vi "Start livestream video from CamServer (TCP CLIENT).vi"(4 "Quality":i32=750 min=0 max=1000, 6 "Resolution":T1 items=["Low", "Med.", "High", "Max."], 7 "Camera":T3="Travcam", 8 "Video name":string, 9 "Video directory path":path, 10 "Write video":bool, 11 "TCP/IP port":u16=80) -> (0 "Error out":errorcluster)   [LabVIEW 2016]
doc: "Starts a video livestream from the camera server. The stream can also be saved to a local directory."
uses:
  Camera enum/Camera enum.ctl
  Camera enum/Camera resolution.ctl
  Anemometry/Anemometry Sub Vis/File/Setup_Filetype.ctl
  <vilib>/vision/Avi.llb/IMAQ AVI2 Refnum.ctl
  Globals/CamServer global.vi
panel:
  in  "Crosshair color":u32(colorbox)=16711935
  in  "Show crosshair":bool=TRUE
  in  "Stop":bool
  out "Video":T2(plugin-control)
  # "PN 25/08/15"
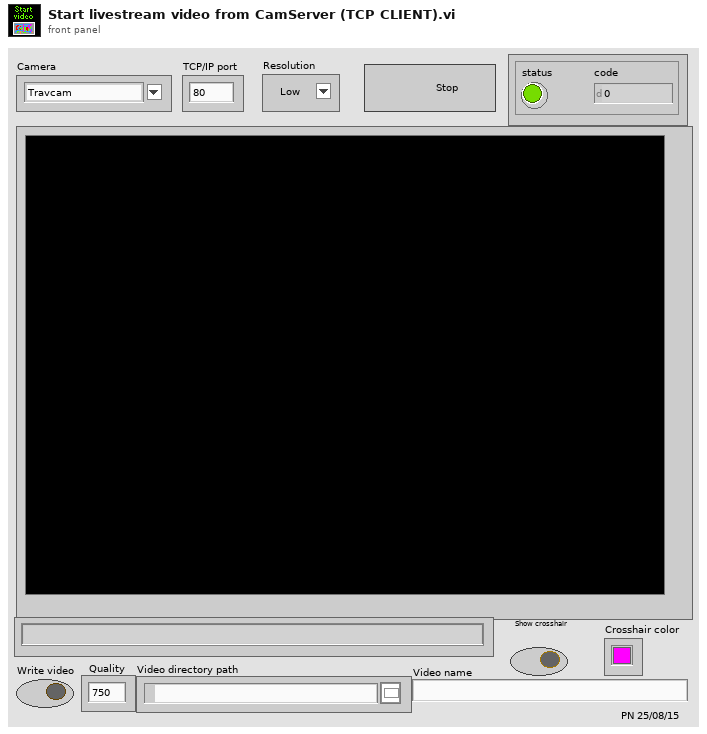
[diagram p1: front panel]
types:
  T1 = typedef "Camera resolution.ctl" = u8
  T2 = typedef "IMAQ Image.ctl" = refnum<image>
  T3 = typedef "Camera enum.ctl" = string
  T4 = typedef "Setup_Filetype.ctl" = enum16{"Measurement Setups", "Calibration Setups", "General", "Results File Plotter Setups", "Speed Calib Tweaks"}
  T5 = typedef "IMAQ AVI2 Refnum.ctl" = refnum<k20>
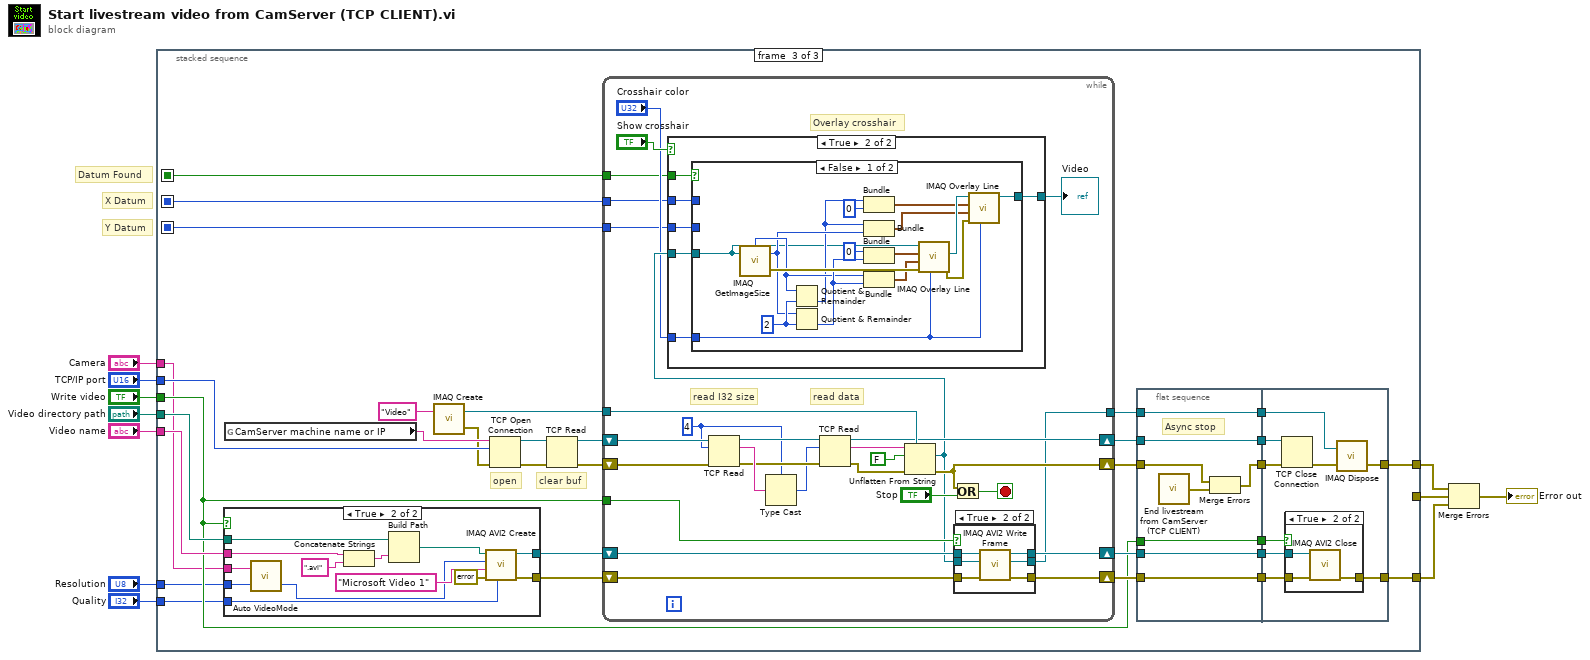
[diagram p0: block diagram]
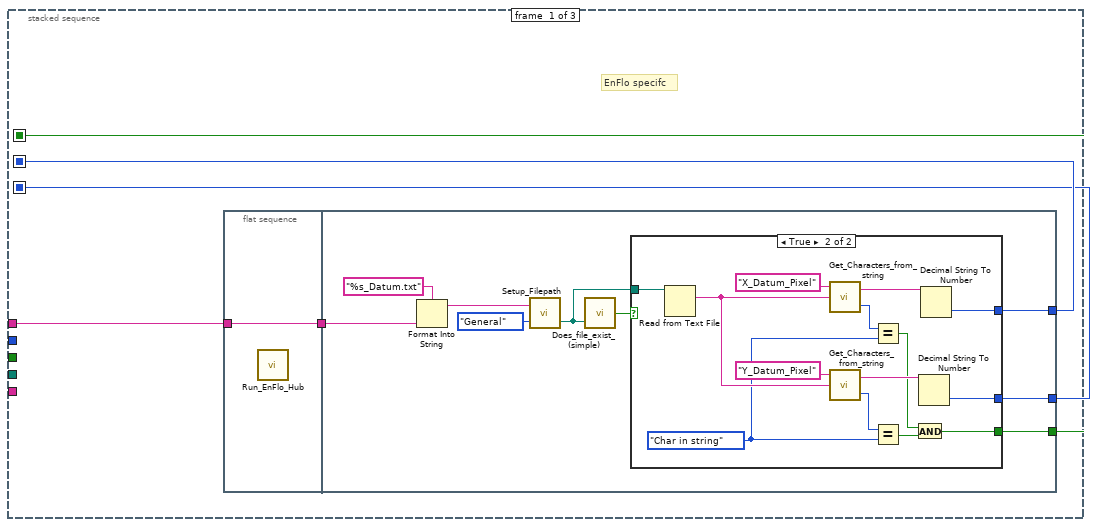
[diagram p2: hidden frame]
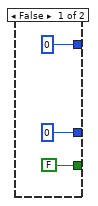
[diagram p3: hidden frame]
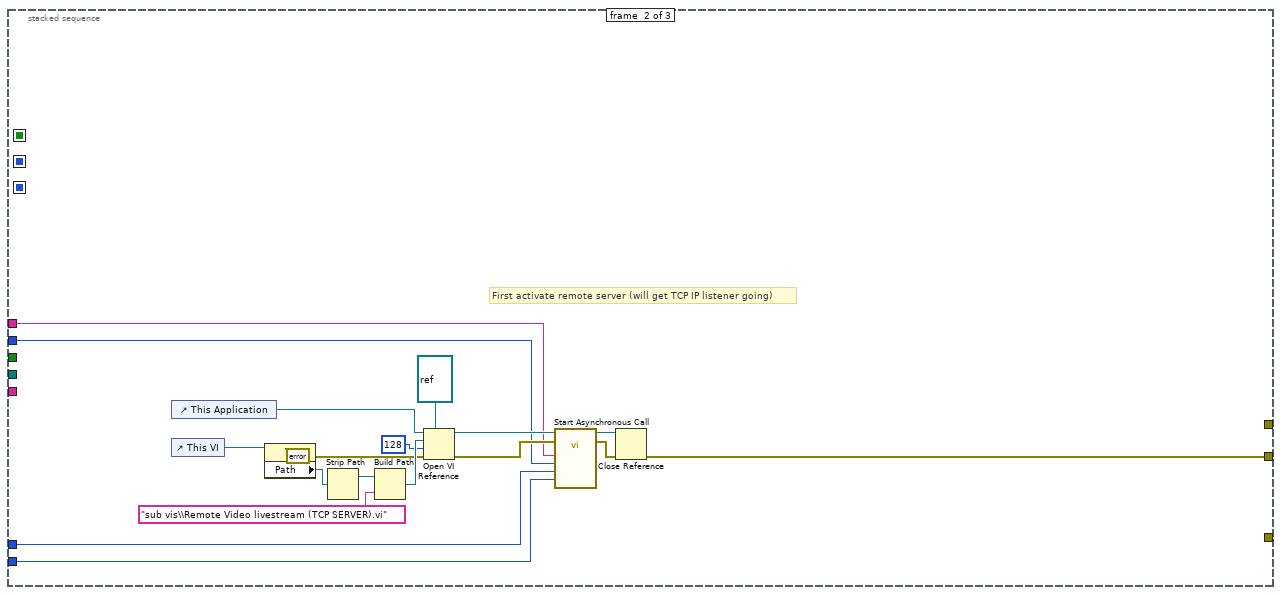
[diagram p4: hidden frame]
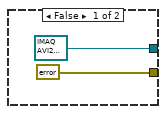
[diagram p5: hidden frame]
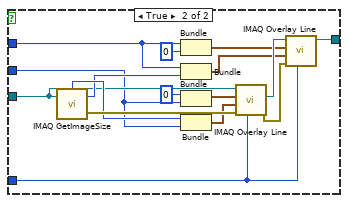
[diagram p8: hidden frame]
diagram:
  # "Datum Found"
  # "Y Datum"
  # "X Datum"
  n1 = stacked-sequence {
    seq-local: [w15 _ _] -> [_ _ w66]
    seq-local: [w14 _ _] -> [_ _ w65]
    seq-local: [w13 _ _] -> [_ _ w67]
    tunnel: "Camera" -> [w16 w48 w64]
    tunnel: "TCP/IP port" -> [_ w47 w95]
    tunnel: "Write video" -> [_ _ w70]
    tunnel: [_ w46 _] -> w8
    tunnel: [_ _ w80] -> w7
    tunnel: [_ _ w73] -> w5
    tunnel: "Video name" -> [_ _ w72]
    tunnel: "Video directory path" -> [_ _ w71]
    tunnel: "Quality" -> [_ w45 w68]
    tunnel: "Resolution" -> [_ w44 w63]
    frame #0 {
      # "EnFlo specifc"
      n2 = flat-sequence {
        tunnel: w16 -> [w17]
        tunnel: [w17] -> w12
        tunnel: [w20] -> w15
        tunnel: [w19] -> w14
        tunnel: [w18] -> w13
        tunnel: w12 -> [w25]
        frame #0 {
          n3 = call "Run_EnFlo_Hub.vi"() -> ()  [unwired: 7 in, 1 out]
        }
        frame #1 {
          n4 = Format Into String(format string="%s_Datum.txt", w25) -> (resulting string=w23:string)  [unwired: 2 in, 1 out]
          n5 = call "Setup_Filepath.vi"("Setup File Type"=Setup_Filetype."General", "Filename in"=w23) -> ("Filename Out"=w21:path)  [unwired: 1 out]
          n6 = call "Does_file_exist_(simple).vi"("Pathname"=w21) -> ("exists?"=w22:bool)
          n7 = case shown="True" w22 {
            tunnel: w21 -> [_ w43]
            tunnel: [0 w40] -> w20
            tunnel: [0 w36] -> w19
            tunnel: [FALSE w30] -> w18
            frame False {
            }
            frame True {
              w35 = enum16{"Char in string", "Char not in string"}."Char in string" ("Status")
              n8 = Read from Text File(file (use dialog)=w43) -> (text=w37:string)  [unwired: 3 in, 3 out]
              n9 = call "Get_Characters_from_string.vi"("Input string"=w37, "Variable name"="X_Datum_Pixel") -> ("Status"=w34:enum16{"Char in string", "Char not in string"}, "Value"=w41:string)  [unwired: 1 in]
              n10 = call "Get_Characters_from_string.vi"("Input string"=w37, "Variable name"="Y_Datum_Pixel") -> ("Status"=w33:enum16{"Char in string", "Char not in string"}, "Value"=w39:string)  [unwired: 1 in]
              n11 = Equal?(x=w34, y=w35) -> (x = y?=w31:bool)
              n12 = Equal?(x=w33, y=w35) -> (x = y?=w32:bool)
              n13 = And(x=w31, y=w32) -> (x .and. y?=w30:bool)
              n14 = Decimal String To Number(string=w39) -> (number=w36:i32)  [unwired: 2 in, 1 out]
              n15 = Decimal String To Number(string=w41) -> (number=w40:i32)  [unwired: 2 in, 1 out]
            }
          }
        }
      }
    }
    frame #1 {
      # "First activate remote server (will get TCP IP listener going)"
      n16 = control-ref of="This Application"() -> (w57:refnum<vi>)
      n17 = control-ref of="This VI"() -> (w62:refnum<vi>)
      n18 = property class="VI"(reference=w62, error in=errorcluster {"status"=FALSE, "code"=0, "source"=""} ("error in (no error)")) -> (error out=w59:errorcluster, "Path"=w55:path)  [unwired: 1 out]
      n19 = Strip Path(path=w55) -> (stripped path=w54:path)  [unwired: 1 out]
      n20 = Build Path(base path=w54, name or relative path="sub vis\\Remote Video livestream (TCP SERVER).vi") -> (appended path=w60:path)
      n21 = Open VI Reference(type specifier VI Refnum (for type only)=refnum<vi> refnum, application reference (local)=w57, vi path=w60, options=128, error in (no error)=w59) -> (vi reference=w53:refnum<vi>, error out=w52:errorcluster)  [unwired: 1 in]
      n22 = call-by-ref "Start Asynchronous Call"(reference=w53, error in=w52, "Quality"=w45, "Resolution"=w44, "TCP/IP port"=w47, "Camera"=w48) -> (reference out=w50:refnum<vi>, error out=w49:errorcluster)  [unwired: 1 out]
      n23 = Close Reference(reference=w50, error in (no error)=w49) -> (error out=w46:errorcluster)
    }
    frame #2 {
      # "open"
      # "clear buf"
      n24 = case shown="True" w70 {
        tunnel: [T5 refnum ("AVI Refnum") w110] -> w79
        tunnel: [errorcluster {"status"=FALSE, "code"=0, "source"=""} ("error out") w109] -> w78
        tunnel: w72 -> [_ w103]
        tunnel: w71 -> [_ w102]
        tunnel: w68 -> [_ w101]
        tunnel: w64 -> [_ w100]
        tunnel: w63 -> [_ w99]
        frame False {
        }
        frame True {
          n25 = call "Auto VideoMode.vi"("Resolution"=w99, "Camera"=w100) -> ("FPS"=w98:u32)  [unwired: 1 out]
          n26 = Concatenate Strings(w103, ".avi" ("name or relative path")) -> (w105:string)
          n27 = Build Path(base path=w102, name or relative path=w105) -> (appended path=w104:path)
          n28 = call "IMAQ AVI2 Create"("Quality"=w101, "error in (no error)"=errorcluster {"status"=FALSE, "code"=0, "source"=""} ("error in"), "Codec"="Microsoft Video 1", "Frames Per Second"=w98, "AVI Path"=w104) -> ("error out"=w109:errorcluster, "AVI Refnum"=w110:T5)  [unwired: 5 in]
        }
      }
      n29 = global read "CamServer global.vi" "CamServer machine name or IP"() -> (w94:string)
      n30 = call "IMAQ Create"("Image Name"="Video") -> ("New Image"=w88:T2, "error out"=w87:errorcluster)  [unwired: 4 in]
      n31 = TCP Open Connection(address=w94, remote port or service name=w95, error in (no error)=w87) -> (connection ID=w92:refnum<k5>, error out=w93:errorcluster)  [unwired: 2 in]
      n32 = TCP Read(connection ID=w92, error in (no error)=w93) -> (connection ID out=w90:refnum<k5>, error out=w91:errorcluster)  [unwired: 3 in, 1 out]
      n33 = while {
        shift-right: [w148] -> w86
        shift-left: w90 -> [w159]
        shift-right: [w147] -> w85
        shift-left: w91 -> [w157]
        tunnel: w88 -> [w150]
        tunnel: [w139] -> w84
        shift-right: [w142] -> w74
        shift-left: w78 -> [w141]
        shift-right: [w143] -> w77
        shift-left: w79 -> [w144]
        tunnel: w70 -> [w140]
        tunnel: w67 -> [w134]
        tunnel: w66 -> [w133]
        tunnel: w65 -> [w132]
        stop <- w145 stop-if-true
        w149 = 4
        # "Overlay crosshair"
        # "read data"
        # "read I32 size"
        n34 = TCP Read(connection ID=w159, bytes to read=w149, error in (no error)=w157) -> (connection ID out=w156:refnum<k5>, data out=w158:string, error out=w155:errorcluster)  [unwired: 2 in]
        n35 = Type Cast(type=w149, x=w158) -> (*(type *) &x=w154:i32)
        n36 = TCP Read(connection ID=w156, bytes to read=w154, error in (no error)=w155) -> (connection ID out=w148:refnum<k5>, data out=w153:string, error out=w151:errorcluster)  [unwired: 2 in]
        n37 = Unflatten From String(type=w150, binary string=w153, data includes array or string size? (T)=FALSE, error in (no error)=w151) -> (value=w137:T2, error out=w147:errorcluster)  [unwired: 1 in, 1 out]
        n38 = case shown="True" "Show crosshair" {
          tunnel: [w160 w166] -> w138
          tunnel: w137 -> [w160 w165]
          tunnel: "Crosshair color" -> [_ w164]
          tunnel: w134 -> [_ w163]
          tunnel: w133 -> [_ w162]
          tunnel: w132 -> [_ w161]
          frame False {
          }
          frame True {
            n39 = case shown="False" w163 {
              tunnel: [w175 w193] -> w166
              tunnel: w165 -> [w168 w187]
              tunnel: w164 -> [w167 w186]
              tunnel: w162 -> [_ w185]
              tunnel: w161 -> [_ w184]
              frame False {
                w182 = 2 ("y")
                n40 = call "IMAQ GetImageSize"("Image"=w168) -> ("Y Resolution"=w170:i32, "X Resolution"=w177:i32, "error out"=w183:errorcluster)  [unwired: 3 in]
                n41 = Quotient & Remainder(x=w177, y=w182) -> (floor(x/y)=w169:i32)  [unwired: 1 out]
                n42 = Quotient & Remainder(x=w170, y=w182) -> (floor(x/y)=w179:i32)  [unwired: 1 out]
                n43 = Bundle(w169, "y"=0) -> (w173:cluster{i32, "y":i32})  [unwired: 1 in]
                n44 = Bundle(w169, "Y Resolution"=w170) -> (w172:cluster{i32, "Y Resolution":i32})  [unwired: 1 in]
                n45 = Bundle("y"=0, w179) -> (w181:cluster{"y":i32, i32})  [unwired: 1 in]
                n46 = Bundle("X Resolution"=w177, w179) -> (w180:cluster{"X Resolution":i32, i32})  [unwired: 1 in]
                n47 = call "IMAQ Overlay Line"("Color"=w167, "error in (no error)"=w183, "End Point"=w180, "Start Point"=w181, "Image"=w168) -> ("error out"=w174:errorcluster, "Image Out"=w176:T2)  [unwired: 5 in]
                n48 = call "IMAQ Overlay Line"("Color"=w167, "error in (no error)"=w174, "End Point"=w172, "Start Point"=w173, "Image"=w176) -> ("Image Out"=w175:T2)  [unwired: 5 in, 1 out]
              }
              frame True {
                n49 = call "IMAQ GetImageSize"("Image"=w187) -> ("Y Resolution"=w188:i32, "X Resolution"=w195:i32, "error out"=w199:errorcluster)  [unwired: 3 in]
                n50 = Bundle(w185, "y"=0) -> (w191:cluster{i32, "y":i32})  [unwired: 1 in]
                n51 = Bundle(w185, "Y Resolution"=w188) -> (w190:cluster{i32, "Y Resolution":i32})  [unwired: 1 in]
                n52 = Bundle("y"=0, w184) -> (w198:cluster{"y":i32, i32})  [unwired: 1 in]
                n53 = Bundle("X Resolution"=w195, w184) -> (w197:cluster{"X Resolution":i32, i32})  [unwired: 1 in]
                n54 = call "IMAQ Overlay Line"("Color"=w186, "error in (no error)"=w199, "End Point"=w197, "Start Point"=w198, "Image"=w187) -> ("error out"=w192:errorcluster, "Image Out"=w194:T2)  [unwired: 5 in]
                n55 = call "IMAQ Overlay Line"("Color"=w186, "error in (no error)"=w192, "End Point"=w190, "Start Point"=w191, "Image"=w194) -> ("Image Out"=w193:T2)  [unwired: 5 in, 1 out]
              }
            }
          }
        }
        "Video" <- w138
        n56 = Or(x=w147, y="Stop") -> (x .or. y?=w145:bool)
        n57 = case shown="True" w140 {
          tunnel: w144 -> [w202 w208]
          tunnel: w137 -> [w200 w207]
          tunnel: [w202 w206] -> w143
          tunnel: [w201 w205] -> w142
          tunnel: w141 -> [w201 w204]
          tunnel: [w200 w203] -> w139
          frame False {
          }
          frame True {
            n58 = call "IMAQ AVI2 Write Frame"("error in (no error)"=w204, "Image"=w207, "AVI Refnum"=w208) -> ("error out"=w205:errorcluster, "Image Out (duplicate)"=w203:T2, "AVI Refnum (duplicate)"=w206:T5)  [unwired: 6 in]
          }
        }
      }
      n59 = flat-sequence {
        tunnel: w84 -> [w117]
        tunnel: w85 -> [w115]
        tunnel: w86 -> [w118]
        tunnel: [w118] -> w83
        tunnel: [w114] -> w82
        tunnel: [w117] -> w81
        tunnel: w77 -> [w113]
        tunnel: [w113] -> w76
        tunnel: w74 -> [w112]
        tunnel: [w112] -> w75
        tunnel: w70 -> [w111]
        tunnel: [w111] -> w69
        tunnel: w83 -> [w127]
        tunnel: w82 -> [w126]
        tunnel: w81 -> [w124]
        tunnel: [w123] -> w80
        tunnel: w76 -> [w122]
        tunnel: w75 -> [w121]
        tunnel: [w120] -> w73
        tunnel: w69 -> [w119]
        frame #0 {
          # "Async stop"
          n60 = call "End livestream from CamServer (TCP CLIENT).vi"() -> ("Error out"=w116:errorcluster)  [unwired: 1 in]
          n61 = Merge Errors(w115, w116) -> (w114:errorcluster)
        }
        frame #1 {
          n62 = TCP Close Connection(connection ID=w127, error in (no error)=w126) -> (error out=w125:errorcluster)  [unwired: 1 in, 1 out]
          n63 = case shown="True" w119 {
            tunnel: w121 -> [w128 w131]
            tunnel: [w128 w130] -> w120
            tunnel: w122 -> [_ w129]
            frame False {
            }
            frame True {
              n64 = call "IMAQ AVI2 Close"("error in (no error)"=w131, "AVI Refnum"=w129) -> ("error out"=w130:errorcluster)  [unwired: 9 in]
            }
          }
          n65 = call "IMAQ Dispose"("Image"=w124, "error in (no error)"=w125) -> ("error out"=w123:errorcluster)  [unwired: 4 in]
        }
      }
    }
  }
  n66 = Merge Errors(w7, w8, w5) -> (→"Error out":errorcluster)
